vi "post_dcs_spot.vi"(8 "error in (no error)":errorcluster, 11 "dcs_spot":T1={"DCS spot ID"=0, "Integer Timestamp"=2, "Spot X"=3.0, "Spot Y"=4.0, "Spot Width X"=0.0, "Spot Width Y"=0.0, "Spot Size"=0, "Experiment Settings ID"=0}) -> (0 "error out":errorcluster)   [LabVIEW 2013]
doc: "Adds a new row to the dcs_spot table."
uses:
  Controls/dcs_spot.ctl
  <vilib>/addons/database/NI_Database_API.lvlib
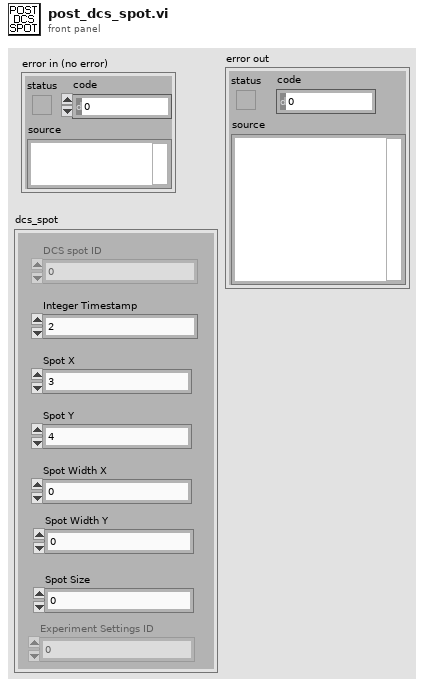
[diagram p1: front panel]
types:
  T1 = typedef "dcs_spot.ctl" = cluster{"DCS spot ID":i32, "Integer Timestamp":i64, "Spot X":dbl, "Spot Y":dbl, "Spot Width X":dbl, "Spot Width Y":dbl, "Spot Size":i32, "Experiment Settings ID":i32}
  T2 = typedef "NI_Database_API.lvlib/Conn ObjectReference.ctl" = refnum<k1>
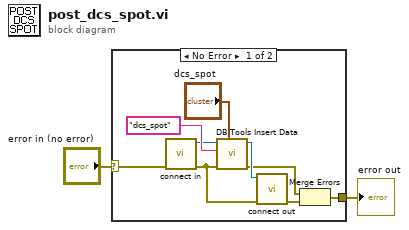
[diagram p0: block diagram]
diagram:
  n1 = case shown="No Error" "error in (no error)" {
    selector: "error in (no error)" -> [w11 w12]
    tunnel: [w3 w12] -> w1
    frame No Error {
      n2 = call "connect in.vi"("error in (no error)"=w11) -> ("error out"=w5:errorcluster, "Database Connection"=w9:T2)  [unwired: 6 in, 1 out]
      n3 = call <vilib>:"DB Tools Insert Data.vi"("data"="dcs_spot", "error in (no error)"=w5, "table"="dcs_spot", "connection reference"=w9) -> ("error out"=w6:errorcluster, "connection reference out"=w8:T2)  [unwired: 6 in]
      n4 = call "connect out.vi"("error in (no error)"=w5, "connection reference"=w8) -> ("error out"=w4:errorcluster)  [unwired: 9 in]
      n5 = Merge Errors(w6, w4) -> (w3:errorcluster)
    }
    frame Error {
    }
  }
  "error out" <- w1
